vi "Event--Drag Ended.vi"(8 "error in":errorcluster, 11 "Selector in":refnum<class "Selector.lvclass">) -> (0 "error out":errorcluster, 3 "Selector out":refnum<class "Selector.lvclass">)   [LabVIEW 2019, in "Selector.lvclass"]
uses:
  Selector.lvclass
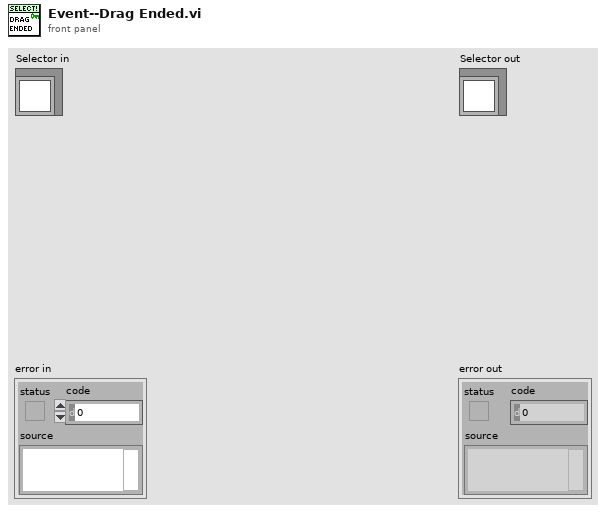
[diagram p1: front panel]
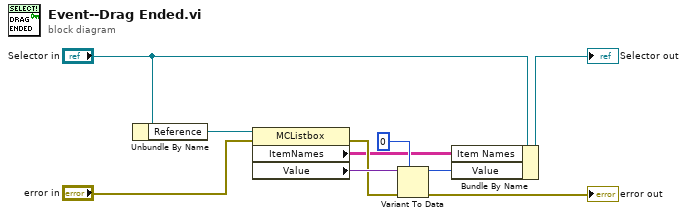
[diagram p0: block diagram]
diagram:
  n1 = Unbundle By Name("Selector in") -> ("Reference"=w10:refnum<vi>)
  n2 = property class="MCListbox"(reference=w10, error in="error in") -> (error out=w4:errorcluster, "ItemNames"=w1:string[][], "Value"=w9:variant)  [unwired: 1 out]
  n3 = Variant To Data(error in=w4, type=0 ("Value"), Variant=w9) -> (data=w6:i32, error out=→"error out":errorcluster)
  n4 = Bundle By Name(cluster="Selector in", "Item Names"=w1, "Value"=w6) -> (→"Selector out":refnum<class "Selector.lvclass">)
